vi "Reset Min-Max.vi"(8 "error in (no error)":errorcluster, 10 "Reset Min/Max (T: Reset)":bool=TRUE, 11 "LS218 in":refnum<class "LS218.lvclass">) -> (0 "error out":errorcluster, 3 "LS218 out":refnum<class "LS218.lvclass">)   [LabVIEW 2013, in "LS218.lvlib" / "LS218.lvclass"]
doc: "This VI resets the minimum and maximum data for all inputs."
uses:
  LS218.lvclass
  LS218.lvclass/LS218.ctl
  <instrlib>/Lake Shore Cryotronics 218/Lake Shore Cryotronics 218.lvlib
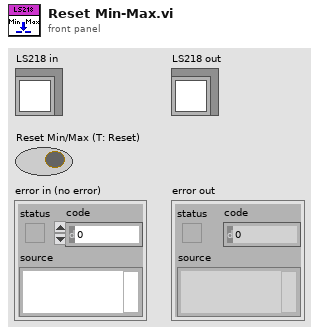
[diagram p1: front panel]
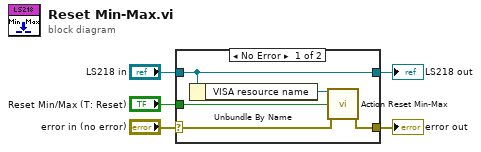
[diagram p0: block diagram]
diagram:
  n1 = case shown="No Error" "error in (no error)" {
    selector: "error in (no error)" -> [w7 w12]
    tunnel: [w6 w12] -> w4
    tunnel: [w10 w11] -> w2
    tunnel: "LS218 in" -> [w10 w11]
    tunnel: "Reset Min/Max (T: Reset)" -> [w8 _]
    frame No Error {
      n2 = Unbundle By Name(w10) -> ("VISA resource name"=w9:refnum<visa-resource-name>)
      n3 = call <instrlib>:"Action Reset Min-Max.vi"("VISA resource name"=w9, "Reset Min/Max (T: Reset)"=w8, "error in (no error)"=w7) -> ("error out"=w6:errorcluster)  [unwired: 11 in, 1 out]
    }
    frame Error {
    }
  }
  "error out" <- w4
  "LS218 out" <- w2
